vi "Update Configure NF Sequence.vi"(8 "error in (no error)":errorcluster, 10 "NF Freq (Hz)":string, 11 "NF in":refnum<class "NF.lvclass">) -> (0 "error out":errorcluster, 3 "NF out":refnum<class "NF.lvclass">)   [LabVIEW 2018, in "NF.lvlib" / "NF.lvclass"]
uses:
  NF.lvclass
  C:/Sequence Automation/Plugins/Measurement Interface.lvlibp/Measurement Interface.lvclass
  NF.lvclass/NF.ctl
  Plugins/Measurement Interface.lvlibp/Private Methods/Active Sequence File/Read Active Sequence File.vi
  Plugins/TestStand API Tools (TSAT).lvlibp/Sequence File Actions/TSAT Sequence File Actions.lvlib
  Plugins/TestStand API Tools (TSAT).lvlibp/TSAT Utilities/TSAT Utilities.lvlib
  Plugins/TestStand API Tools (TSAT).lvlibp/Sequence Actions/TSAT Sequence Actions.lvlib
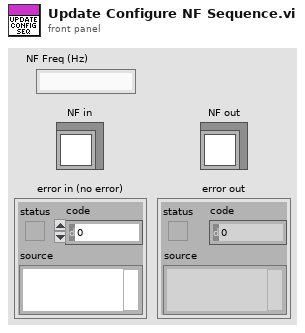
[diagram p1: front panel]
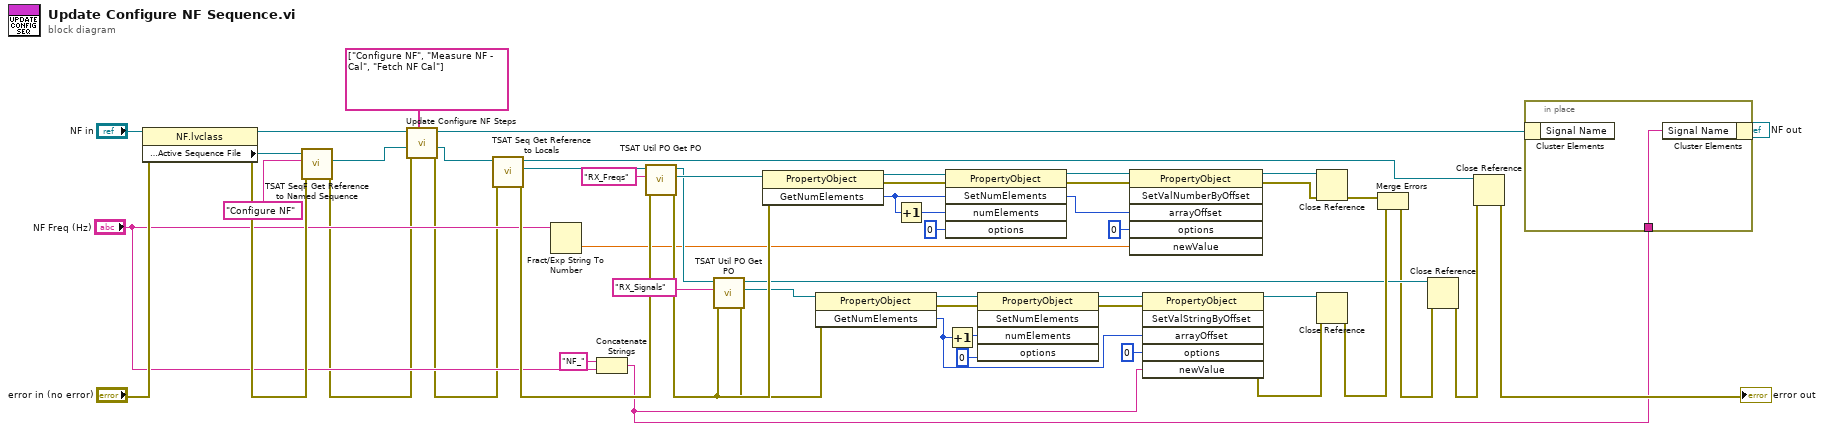
[diagram p0: block diagram]
diagram:
  n1 = property class="NF.lvclass"(reference="NF in", error in="error in (no error)") -> (reference out=w10:refnum<class "NF.lvclass">, error out=w50:errorcluster, "Protected Methods:Active Sequence File"=w51:refnum<k7>)
  n2 = call "TSAT SeqF Get Reference to Named Sequence.vi"("Error In"=w50, "Seqeunce to Retrieve"="Configure NF", "Sequence File In"=w51) -> ("Error Out"=w8:errorcluster, "Named Sequence"=w7:refnum<k7>)  [unwired: 6 in, 1 out]
  n3 = call-dynamic "Update Configure NF Steps.vi"("Steps to Update"=string[] ["Configure NF", "Measure NF - Cal", "Fetch NF Cal"], "error in (no error)"=w8, "Configure NF Sequence Ref"=w7, "NF in"=w10) -> ("error out"=w5:errorcluster, "Configure NF Sequence Ref"=w6:refnum<k7>, "NF out"=w9:refnum<class "NF.lvclass">)  [unwired: 5 in]
  n4 = call "TSAT Seq Get Reference to Locals.vi"("Error In"=w5, "Sequence In"=w6) -> ("Error Out"=w43:errorcluster, "Locals"=w45:refnum<k7>, "Sequence Out"=w11:refnum<k7>)  [unwired: 7 in]
  n5 = Fract/Exp String To Number(string="NF Freq (Hz)") -> (number=w28:dbl)  [unwired: 3 in, 1 out]
  n6 = Concatenate Strings("NF_" ("string"), "NF Freq (Hz)") -> (w25:string)
  n7 = call "TSAT Util PO Get PO.vi"("error in (no error)"=w43, "Sub Property to Retrieve"="RX_Freqs", "Property Object in"=w45) -> ("error out"=w41:errorcluster, "SubProperty"=w46:refnum<k7>, "PropertyObjectOut"=w42:refnum<k7>)  [unwired: 6 in]
  n8 = call "TSAT Util PO Get PO.vi"("error in (no error)"=w41, "Sub Property to Retrieve"="RX_Signals", "Property Object in"=w42) -> ("error out"=w39:errorcluster, "SubProperty"=w40:refnum<k7>, "PropertyObjectOut"=w3:refnum<k7>)  [unwired: 6 in]
  n9 = invoke class="PropertyObject" method="GetNumElements"(reference=w46, error in=w41) -> (reference out=w22:refnum<k7>, error out=w44:errorcluster, "GetNumElements"=w20:i32)  [unwired: 1 in]
  n10 = invoke class="PropertyObject" method="GetNumElements"(reference=w40, error in=w39) -> (reference out=w16:refnum<k7>, error out=w38:errorcluster, "GetNumElements"=w14:i32)  [unwired: 1 in]
  n11 = Increment(x=w20) -> (x+1=w19:i32)
  n12 = invoke class="PropertyObject" method="SetNumElements"(reference=w22, error in=w44, "numElements"=w19, "options"=0) -> (reference out=w21:refnum<k7>, error out=w23:errorcluster)  [unwired: 1 in, 3 out]
  n13 = Increment(x=w14) -> (x+1=w13:i32)
  n14 = invoke class="PropertyObject" method="SetNumElements"(reference=w16, error in=w38, "numElements"=w13, "options"=0) -> (reference out=w15:refnum<k7>, error out=w17:errorcluster)  [unwired: 1 in, 3 out]
  n15 = invoke class="PropertyObject" method="SetValNumberByOffset"(reference=w21, error in=w23, "arrayOffset"=w20, "options"=0, "newValue"=w28) -> (reference out=w37:refnum<k7>, error out=w36:errorcluster)  [unwired: 1 in, 4 out]
  n16 = invoke class="PropertyObject" method="SetValStringByOffset"(reference=w15, error in=w17, "arrayOffset"=w14, "options"=0, "newValue"=w25) -> (reference out=w35:refnum<k7>, error out=w34:errorcluster)  [unwired: 1 in, 4 out]
  n17 = Close Reference(reference=w37, error in (no error)=w36) -> (error out=w33:errorcluster)
  n18 = Close Reference(reference=w35, error in (no error)=w34) -> (error out=w32:errorcluster)
  n19 = Merge Errors(w33, w32) -> (w2:errorcluster)
  n20 = Close Reference(reference=w3, error in (no error)=w2) -> (error out=w1:errorcluster)
  n21 = Close Reference(reference=w11, error in (no error)=w1) -> (error out=→"error out":errorcluster)
  n22 = in-place {
    in-place-border: w25 -> [w54]
    n23 = in-place-cluster #1(w9) -> ()  [unwired: 1 out]
    n24 = in-place-cluster #1("Signal Name"=w54) -> (→"NF out":refnum<class "NF.lvclass">)
  }
